vi "fgt get valve Channels Info.vi"(8 "error in (no error)":errorcluster) -> (0 "error out":errorcluster, 2 "Valve channels type":T1[](array[typedef]), 3 "Valve channels info":T2[](array[typedef]) {"indexID" format="%.0x"; "index" format="%.0x"; "position" format="%.0x"; "DeviceSN" format="%.0x"; "firmware" format="%.0x"; "ControllerSN" format="%.0x"})   [LabVIEW 2020, in "fgt_SDK.lvlib"]
doc: "Retrieve information about each initialized sensor channel. This function is useful in order to get channels order, controller, unique ID and InstrType.\nBy default this array is built with FRP Flow Units first, followed by Flow EZ Flow Units, followed by IPS modules. If only one instrument is used, index is the default channel indexing starting at 0.\nYou can initialize instruments in specific order using fgt_initEx function"
uses:
  fgt_SDK.lvlib
  TypeDefs/fgt_CHANNEL_INFO.ctl
  TypeDefs/fgt_INSTRUMENT_TYPE.ctl
  TypeDefs/fgt_VALVE_TYPE.ctl
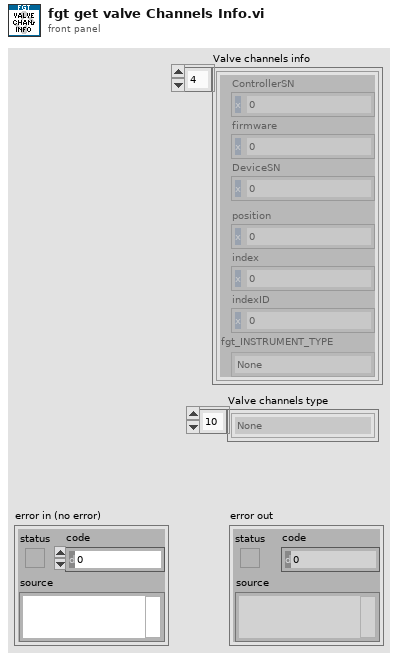
[diagram p1: front panel]
types:
  T1 = typedef "fgt_SDK.lvlib/fgt_VALVE_TYPE.ctl" = enum32{"None", "MSwitch", "TwoSwitch", "LSwitch", "PSwitch"}
  T2 = typedef "fgt_SDK.lvlib/fgt_CHANNEL_INFO.ctl" = cluster{"ControllerSN":u16, "firmware":u16, "DeviceSN":u16, "position":u32, "index":u32, "indexID":u32, "fgt_INSTRUMENT_TYPE":T3}
  T3 = typedef "fgt_SDK.lvlib/fgt_INSTRUMENT_TYPE.ctl" = enum32{"None", "MFCS", "MFCS_EZ", "FRP", "LineUP", "IPS"}
  T4 = cluster{"ControllerSN":u16, "firmware":u16, "DeviceSN":u16, "Padding":u16, "position":u32, "index":u32, "indexID":u32, "fgt_INSTRUMENT_TYPE":T3}
  T5 = cluster{"ControllerSN":u16, "firmware":u16, "DeviceSN":u16, "Padding":u16, "position":u32, "index":u32, "indexID":u32, "fgt_INSTRUMENT_TYPE":T3}[]
  T6 = typedef "fgt_SDK.lvlib/fgt_STATUS_INFO.ctl" = cluster{"InstrType":T3, "instrSN":u16, "errorCode":u8, "infoCode":u8, "detail":string}
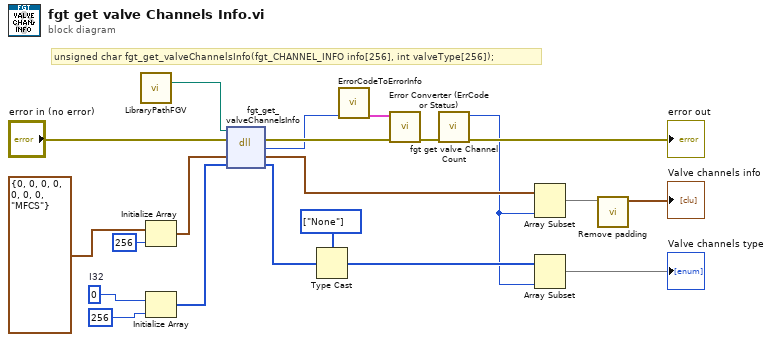
[diagram p0: block diagram]
diagram:
  w12 = T1[] [enum."None"] items=["None", "MSwitch", "TwoSwitch", "LSwitch", "PSwitch"]
  w14 = 0  # I32
  # "unsigned char fgt_get_valveChannelsInfo(fgt_CHANNEL_INFO info[256], int valveType[256]);"
  n1 = call "LibraryPathFGV.vi"() -> ("Path Out"=w1:path)  [unwired: 14 in, 1 out]
  n2 = Initialize Array(T4 {"ControllerSN"=0, "firmware"=0, "DeviceSN"=0, "Padding"=0, "position"=0, "index"=0, "indexID"=0, "fgt_INSTRUMENT_TYPE"=enum."MFCS"} ("fgt_CHANNEL_INFO"), 256 ("dimension size")) -> (w16:T5)
  n3 = Initialize Array(w14, 256 ("dimension size")) -> (w13:i32[])
  n4 = dll-call lib="C:/Workspace/fgt-SDK/LabVIEW/dlls/fgt_SDK_*.*" fn="fgt_get_valveChannelsInfo"(path in=w1, error in="error in (no error)", "info"=w16, "valveType"=w13) -> (error out=w20:errorcluster, "return type"=w19:u8, "info"=w9:T5, "valveType"=w11:i32[])  [unwired: 1 in, 1 out]
  n5 = Type Cast(type=w12, x=w11) -> (*(type *) &x=w10:T1[])
  n6 = call "ErrorCodeToErrorInfo.vi"("return type"=w19) -> ("StatusInfo"=w18:T6)  [unwired: 10 in]
  n7 = call "Error Converter (ErrCode or Status).vi"("error in (no error)"=w20, "StatusInfo"=w18) -> ("error out"=w4:errorcluster)  [unwired: 9 in]
  n8 = call "fgt get valve Channel Count.vi"("error in (no error)"=w4) -> ("error out"=→"error out":errorcluster, "nbVChan out"=w2:u32)  [unwired: 9 in]
  n9 = Array Subset(array=w9, length=w2) -> (w6:T5)  [unwired: 1 in]
  n10 = Array Subset(array=w10, length=w2) -> (→"Valve channels type":T1[])  [unwired: 1 in]
  n11 = call "Remove padding.vi"("Array in"=w6) -> ("Array out"=→"Valve channels info":T2[])  [unwired: 10 in]
